vi "Convert Time to H_M_S.vi"(7 "Initial Scan Location":u32, 8 "error in":errorcluster, 10 "Tot. Timer Format":u16, 11 "Time Data String":string="Time Data String") -> (0 "error out":errorcluster, 1 "[sec]":dbl, 2 "[min]":dbl, 3 "[hr]":dbl, 5 "Offset Past Scan":u32)   [LabVIEW 2018]
doc: "Converts the Totalizer Timer data string into H:M:S doubles based on the time string format. A timer format of 2 is used if the Totalizer Timer is already outputting data in the H:M:S format.\n\nIf unsure of the format your Alicat uses, the output of the \"Read Measurement Format\" sub-VI will output the timer format for use with this sub-VI."
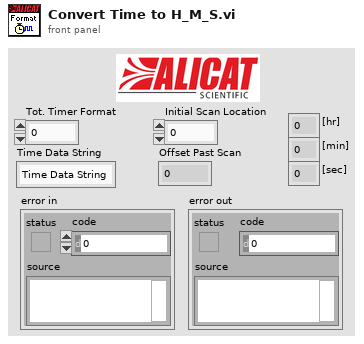
[diagram p1: front panel]
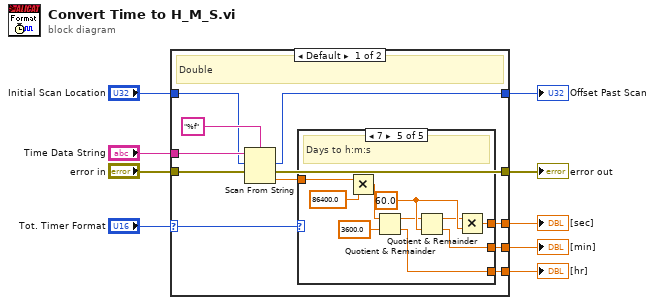
[diagram p0: block diagram]
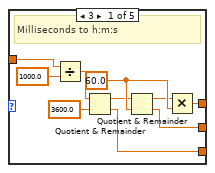
[diagram p2: hidden frame]
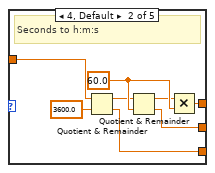
[diagram p3: hidden frame]
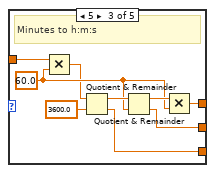
[diagram p4: hidden frame]
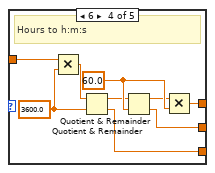
[diagram p5: hidden frame]
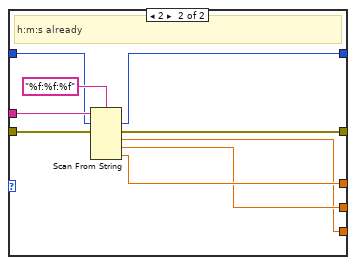
[diagram p6: hidden frame]
diagram:
  n1 = case shown="Default" "Tot. Timer Format" {
    selector: "Tot. Timer Format" -> [w18 _]
    tunnel: "Time Data String" -> [w20 w75]
    tunnel: "error in" -> [w12 w73]
    tunnel: [w13 w72] -> w7
    tunnel: [w16 w71] -> w3
    tunnel: [w15 w70] -> w4
    tunnel: [w14 w69] -> w5
    tunnel: [w10 w68] -> w2
    tunnel: "Initial Scan Location" -> [w11 w67]
    frame Default {
      # "Double"
      n2 = Scan From String(format string="%f", input string=w20, initial scan location=w11, error in=w12) -> (offset past scan=w10:u32, error out=w13:errorcluster, output 1=w17:dbl)  [unwired: 1 in, 1 out]
      n3 = case shown="7" w18 {
        tunnel: w17 -> [w29 w31 w41 w49 w65]
        tunnel: [w23 w34 w44 w51 w60] -> w16
        tunnel: [w22 w33 w43 w53 w59] -> w15
        tunnel: [w21 w32 w42 w52 w58] -> w14
        frame 3 {
          w28 = 60.0 ("y")
          # "Milliseconds to h:m:s"
          n4 = Divide(x=w29, y=1000.0) -> (x/y=w24:dbl)
          n5 = Quotient & Remainder(x=w24, y=3600.0) -> (x-y*floor(x/y)=w26:dbl, floor(x/y)=w21:dbl)
          n6 = Quotient & Remainder(x=w26, y=w28) -> (x-y*floor(x/y)=w27:dbl, floor(x/y)=w22:dbl)
          n7 = Multiply(x=w27, y=w28) -> (x*y=w23:dbl)
        }
        frame 4, Default {
          w38 = 60.0 ("y")
          # "Seconds to h:m:s"
          n8 = Quotient & Remainder(x=w31, y=3600.0) -> (x-y*floor(x/y)=w36:dbl, floor(x/y)=w32:dbl)
          n9 = Quotient & Remainder(x=w36, y=w38) -> (x-y*floor(x/y)=w37:dbl, floor(x/y)=w33:dbl)
          n10 = Multiply(x=w37, y=w38) -> (x*y=w34:dbl)
        }
        frame 5 {
          w40 = 60.0 ("y")
          # "Minutes to h:m:s"
          n11 = Multiply(x=w41, y=w40) -> (x*y=w39:dbl)
          n12 = Quotient & Remainder(x=w39, y=3600.0) -> (x-y*floor(x/y)=w46:dbl, floor(x/y)=w42:dbl)
          n13 = Quotient & Remainder(x=w46, y=w40) -> (x-y*floor(x/y)=w47:dbl, floor(x/y)=w43:dbl)
          n14 = Multiply(x=w47, y=w40) -> (x*y=w44:dbl)
        }
        frame 6 {
          w56 = 60.0 ("y")
          w48 = 3600.0 ("y")
          # "Hours to h:m:s"
          n15 = Multiply(x=w49, y=w48) -> (x*y=w50:dbl)
          n16 = Quotient & Remainder(x=w50, y=w48) -> (x-y*floor(x/y)=w54:dbl, floor(x/y)=w52:dbl)
          n17 = Quotient & Remainder(x=w54, y=w56) -> (x-y*floor(x/y)=w55:dbl, floor(x/y)=w53:dbl)
          n18 = Multiply(x=w55, y=w56) -> (x*y=w51:dbl)
        }
        frame 7 {
          w64 = 60.0 ("y")
          # "Days to h:m:s"
          n19 = Multiply(x=w65, y=86400.0) -> (x*y=w57:dbl)
          n20 = Quotient & Remainder(x=w57, y=3600.0) -> (x-y*floor(x/y)=w62:dbl, floor(x/y)=w58:dbl)
          n21 = Quotient & Remainder(x=w62, y=w64) -> (x-y*floor(x/y)=w63:dbl, floor(x/y)=w59:dbl)
          n22 = Multiply(x=w63, y=w64) -> (x*y=w60:dbl)
        }
      }
    }
    frame 2 {
      # "h:m:s already"
      n23 = Scan From String(format string="%f:%f:%f", input string=w75, initial scan location=w67, error in=w73) -> (offset past scan=w68:u32, error out=w72:errorcluster, output 1=w69:dbl, output 2=w70:dbl, output 3=w71:dbl)  [unwired: 3 in, 1 out]
    }
  }
  "error out" <- w7
  "[hr]" <- w5
  "[min]" <- w4
  "[sec]" <- w3
  "Offset Past Scan" <- w2
